vi "UserManagement.vi"() -> ()   [LabVIEW 2011]
uses:
  System.Windows.Forms
  System.Data
panel:
  in  "取消按钮":bool
  in  "DataGridView":refnum<k24>(container)
  in  "确定按钮":bool
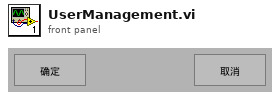
[diagram p1: front panel]
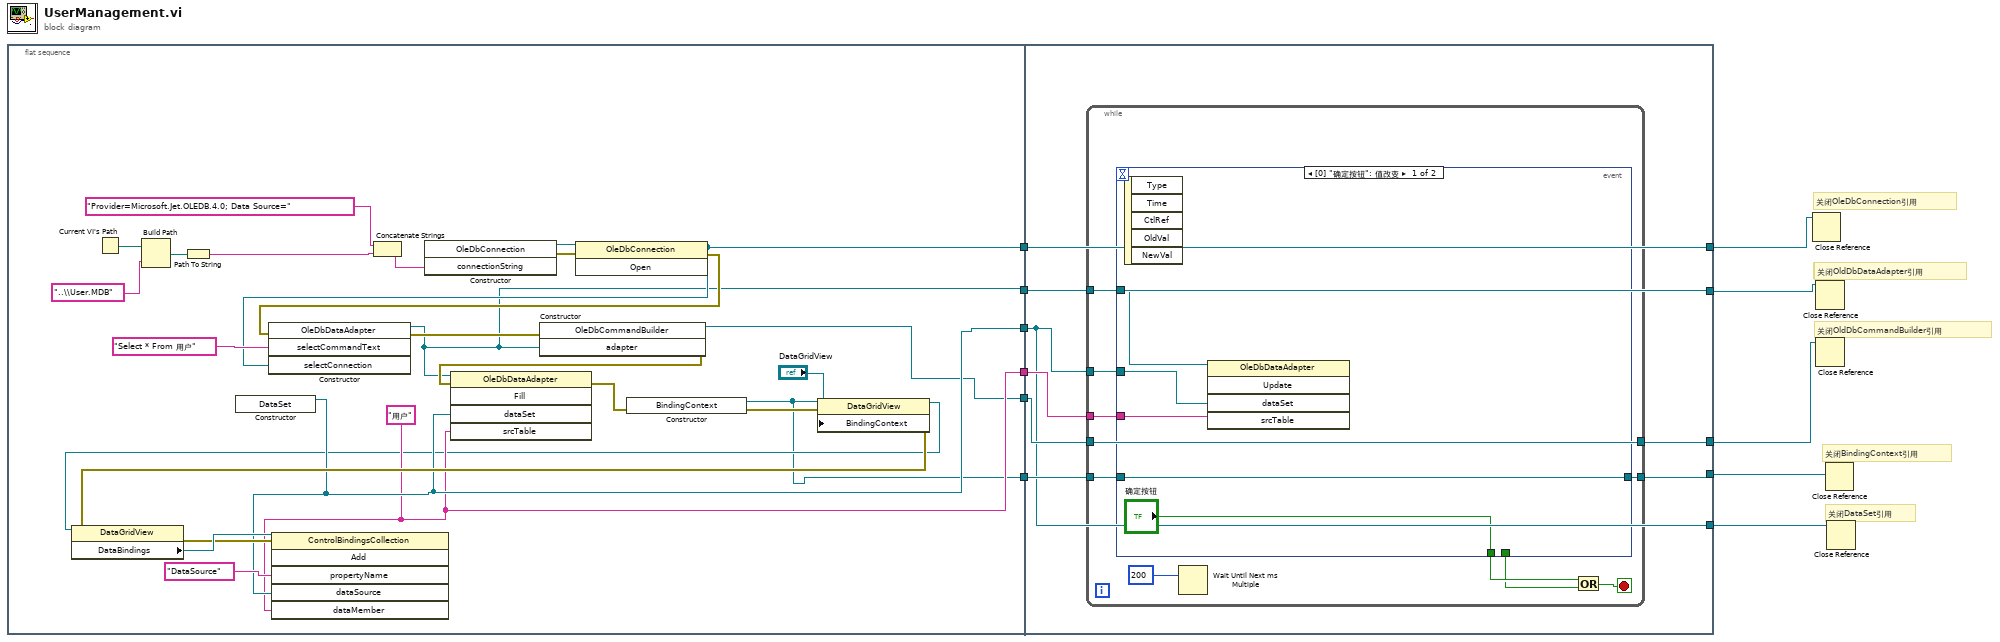
[diagram p0: block diagram]
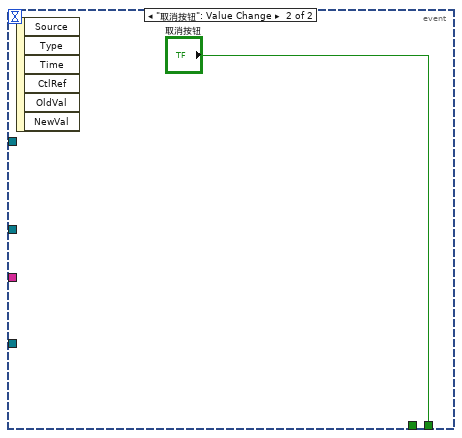
[diagram p2: hidden frame]
diagram:
  # "关闭DataSet引用"
  # "关闭BindingContext引用"
  # "关闭OldDbCommandBuilder引用"
  # "关闭OldDbDataAdapter引用"
  # "关闭OldDbDataAdapter引用"
  # "关闭OleDbConnection引用"
  n1 = flat-sequence {
    tunnel: [w22] -> w11
    tunnel: [w21] -> w10
    tunnel: [w15] -> w9
    tunnel: [w14] -> w8
    tunnel: [w13] -> w7
    tunnel: [w12] -> w3
    tunnel: w11 -> [w39]
    tunnel: w10 -> [w45]
    tunnel: w9 -> [w43]
    tunnel: w8 -> [w38]
    tunnel: w7 -> [w44]
    tunnel: [w43] -> w6
    tunnel: [w38] -> w5
    tunnel: [w42] -> w4
    tunnel: w3 -> [w41]
    tunnel: [w40] -> w2
    tunnel: [w39] -> w1
    frame #0 {
      w21 = "用户" ("srcTable")
      n2 = Current VI's Path() -> (path=w17:path)
      n3 = Build Path(base path=w17, name or relative path="..\\User.MDB" ("名称或相对路径")) -> (appended path=w18:path)
      n4 = Path To String(path=w18) -> (string=w16:string)
      n5 = constructor class="DataSet"() -> (reference out=w22:refnum<k24>)  [unwired: 3 in, 2 out]
      n6 = Concatenate Strings("Provider=Microsoft.Jet.OLEDB.4.0; Data Source=" ("字符串"), w16) -> (w36:string)
      n7 = constructor class="OleDbConnection"("connectionString"=w36) -> (reference out=w35:refnum<k24>, error out=w34:errorcluster)  [unwired: 3 in, 2 out]
      n8 = invoke class="OleDbConnection" method="Open"(reference=w35, error in=w34) -> (reference out=w15:refnum<k24>, error out=w32:errorcluster)  [unwired: 1 in, 1 out]
      n9 = constructor class="OleDbDataAdapter"(error in=w32, "selectCommandText"="Select * From 用户", "selectConnection"=w15) -> (reference out=w14:refnum<k24>, error out=w31:errorcluster)  [unwired: 2 in, 3 out]
      n10 = constructor class="OleDbCommandBuilder"(error in=w31, "adapter"=w14) -> (reference out=w13:refnum<k24>, error out=w30:errorcluster)  [unwired: 2 in, 2 out]
      n11 = invoke class="OleDbDataAdapter" method="Fill"(reference=w14, error in=w30, "dataSet"=w22, "srcTable"=w21) -> (error out=w29:errorcluster)  [unwired: 1 in, 4 out]
      n12 = constructor class="BindingContext"(error in=w29) -> (reference out=w12:refnum<k24>, error out=w27:errorcluster)  [unwired: 2 in, 1 out]
      n13 = property class="DataGridView"(reference="DataGridView", error in=w27, "BindingContext"=w12) -> (reference out=w20:refnum<k24>, error out=w24:errorcluster)
      n14 = property class="DataGridView"(reference=w20, error in=w24) -> (error out=w23:errorcluster, "DataBindings"=w26:refnum<k24>)  [unwired: 1 out]
      n15 = invoke class="ControlBindingsCollection" method="Add"(reference=w26, error in=w23, "propertyName"="DataSource", "dataSource"=w22, "dataMember"=w21) -> ()  [unwired: 1 in, 6 out]
    }
    frame #1 {
      n16 = while {
        tunnel: w39 -> [w51]
        tunnel: w45 -> [w50]
        tunnel: w44 -> [w49]
        tunnel: [w49] -> w42
        tunnel: w41 -> [w48]
        tunnel: [w47] -> w40
        tunnel: w38 -> [w46]
        stop <- w54 stop-if-true
        n17 = event shown="[0] \"确定按钮\": 值改变" {
          selector: _ -> [_ _]
          dyn-events: _ -> [_ _]
          timeout: _ -> [_ _]
          tunnel: ["确定按钮" _] -> w53
          tunnel: [_ "取消按钮"] -> w52
          tunnel: w51 -> [w59 _]
          tunnel: w50 -> [w58 _]
          tunnel: w48 -> [w57 _]
          tunnel: [w57 _] -> w47
          tunnel: w46 -> [w56 _]
          event "确定按钮": Value Change {
            n18 = event-data() -> ()  [unwired: 1 in, 5 out]
            n19 = invoke class="OleDbDataAdapter" method="Update"(reference=w56, "dataSet"=w59, "srcTable"=w58) -> ()  [unwired: 2 in, 5 out]
          }
          event "取消按钮": Value Change {
            n20 = event-data() -> ()  [unwired: 1 in, 6 out]
          }
        }
        n21 = Wait Until Next ms Multiple(millisecond multiple=u32 200 ("毫秒计时值")) -> ()  [unwired: 1 out]
        n22 = Or(x=w53, y=w52) -> (x .or. y?=w54:bool)
      }
    }
  }
  n23 = Close Reference(reference=w6) -> ()  [unwired: 1 in, 1 out]
  n24 = Close Reference(reference=w5) -> ()  [unwired: 1 in, 1 out]
  n25 = Close Reference(reference=w4) -> ()  [unwired: 1 in, 1 out]
  n26 = Close Reference(reference=w2) -> ()  [unwired: 1 in, 1 out]
  n27 = Close Reference(reference=w1) -> ()  [unwired: 1 in, 1 out]
